vi "Brk_Pt_PRF.vi"(0 "Motion Settings In":T1={"No Motion?"=FALSE, "Motion System"=enum."NI 735x", "Motion Bd ID"=1, "Motion Profile"="SMAC1", "# Axis"=1, "Reverse Z axis?"=TRUE, "SMAC Axis"=0, "scan pair"=enum."y-(x) scan", "RT fps"=6.0, "Steps per mm"=[1000, 1000, 1000, 1000], "Motor Parameters"={"velocity ct/s"=[10000.0, 10000.0, 10000.0, 50000.0], "accel ct/s^2"=[50000.0, 50000.0, 50000.0, 200000.0]}, "One Way Scan"=FALSE, "Reverse One Way Scan"=FALSE, "Global Position (mm)"=[], "Plane"=0, "Distance between\nscan lines (um)"=0.0, "Distance between\nscan planes (um)"=0.0, "number of scan planes"=1, "Total steps in line"=0, "Xtra plane\ndistance  (um)"=100, "Xtra planes "=1, "Add Axis"=FALSE, "overshoot cts"=200, "BKPT Shift"=0, "Scan Start Time (ms)"=0, "ESP VISA"="GPIB::1::INSTR", "3rd Axis"=1, "GL Ref Out"=refnum, "Galil Address"=""} {"3rd Axis" items=["x", "y", "z", "w"]; "Xtra planes" min=1; "Xtra plane\ndistance  (um)" min=0; "Distance between\nscan planes (um)" format="%.2f"; "Distance between\nscan lines (um)" format="%.2f"; "SMAC Axis" items=["None"=0, "Axis 1"=1, "Axis 2"=2, "Axis 3"=3, "Axis 4"=4, "Axis 5"=5, "Axis 6"=6, "Axis 7"=7, "Axis 8"=8, "Vector Space 1"=17, "Vector Space 2"=18, "Vector Space 3"=19, "Vector Space 4"=20]; "Motion Bd ID" min=1 max=32 step=1}, 1 "Axis":u16(ring)=1 items=["Axis 1"=1, "Axis 2"=2, "Axis 3"=3, "Axis 4"=4, "Axis 5"=5, "Axis 6"=6, "Axis 7"=7, "Axis 8"=8], 2 "Reverse ?":bool, 11 "error in (no error)":errorcluster, 13 "Offset":i32) -> (4 "Start Position":i32, 6 "End Position":i32, 10 "Motion error":bool)   [LabVIEW 2022 SP3]
doc: "EXAMPLE: DO_WHILE Loop (Onboard Programming Template)\n\nSUMMARY:\nThis FlexMotion example demonstrates the implementation of a DO_WHILE loop data structure in an onboard program. The C equivalent of the data structure implemented here is:\n\ndo {\n// code to be repeated\nloopVar = loopVar - increment;\n} while (loopVar != 0);\n\nTHEORY OF OPERATION:\nThe flow of the DO_WHILE loop data structure goes as follows:\n(1) Program storage is begun.\n(2) The DO_WHILE loop is set up. (Loop Variable and Increment are each defined and initialized.)\n(3) A code delimiter is set using label #1.\n(4) Code to be executed each time through loop is run (in the template program, the loop variable is decremented).\n(5) The loop variable or other test condition is checked.\n(6) If the test condition is true, then we jump back to label #1. Otherwise, the condition is false so the loop terminates.\n(7) Program storage is ended.\n\nDEVELOPMENT DETAILS:\nApplication Software: LabVIEW 5.0.x\nHardware: FlexMotion controller\nDriver Software: FlexMotion Software 4.0\n\nREQUIRED HARDWARE:\n(controller only)\n\nINSTRUCTIONS:\n(0) Initialize the FlexMotion controller before running this VI. \n(1) Add the FlexMotion functions you want to execute into the block diagram where noted.\n(2) Run the VI to store the program. (The program will not be executed at this time.)\n(3) You can then run the program you have stored by calling the run_prog.flx function with the appropriate program number.\n\nADDITIONAL NOTES:\n(a) You should read the following items before writing FlexMotion onboard programs:\n(1) The Onboard Programs section of the FlexMotion Hardware User Manual (page 4-9 in the November 1998 edition).\n(2) The section about onboard variables in your FlexMotion Software Reference Manual (pages 4-11 and 4-12 in the November 1998 edition)\n(3) You will find the chapter of the FlexMotion Software Reference Manual concerning the Onboard Programming functions to be an invaluable reference resource (Chapter 12 of the November 1998 edition) along with the online help for the VI functions.\n(b) This template repeats the DO_WHILE loop as long as an expression with a variable evaluates to be true. However, you may evaluate other conditions such as move complete status instead.\n\n*NOTE: This example is not supported on the 7334 controller."
uses:
  MotionParameters.ctl
  MotionSys.ctl
  -MotionRoutines/ScanAxis.ctl
  -MotionRoutines/3rdAxis.ctl
  <vilib>/Motion/FlexMotion/FunctionsVIs/Trajectory.llb/Load Acceleration/Deceleration.flx
  <vilib>/Motion/FlexMotion/FunctionsVIs/StartStopMotion.llb/Start Motion (8 axes).flx
  <vilib>/Motion/FlexMotion/FunctionsVIs/Trajectory.llb/Wait for Move Complete (8 axes).flx
  Pulsers/PulserGlobals.vi
panel:
  out "Motion stop loop":i32
  # "Doesn't seem to work. Too much overhead to maintain PRF"
  # "1-D and 2-D B scan settings"
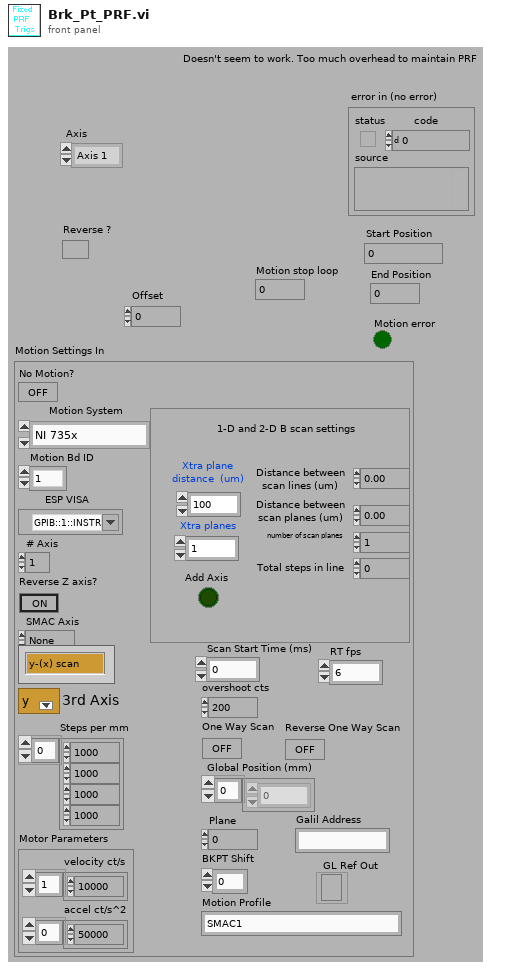
[diagram p1: front panel]
types:
  T1 = typedef "MotionParameters.ctl" = cluster{"No Motion?":bool, "Motion System":T2, "Motion Bd ID":u8, "Motion Profile":string, "# Axis":i8, "Reverse Z axis?":bool, "SMAC Axis":u16, "scan pair":T3, "RT fps":sgl, "Steps per mm":i32[], "Motor Parameters":cluster{"velocity ct/s":dbl[], "accel ct/s^2":dbl[]}, "One Way Scan":bool, "Reverse One Way Scan":bool, "Global Position (mm)":dbl[], "Plane":i32, "Distance between\nscan lines (um)":sgl, "Distance between\nscan planes (um)":sgl, "number of scan planes":i32, "Total steps in line":i32, "Xtra plane\ndistance  (um)":i32, "Xtra planes ":i32, "Add Axis":bool, "overshoot cts":i32, "BKPT Shift":i32, "Scan Start Time (ms)":u32, "ESP VISA":refnum<visa-resource-name>, "3rd Axis":T4, "GL Ref Out":refnum<k7>, "Galil Address":string}
  T2 = typedef "MotionSys.ctl" = enum16{"MM3000", "NI 735x", "Newport ESP", "No Motion Card", "Galil"}
  T3 = typedef "ScanAxis.ctl" = enum16{"y-(x) scan", "x-(y) scan", "z-(x) scan", "z-(y) scan", "y-(z) scan", "x-(z) scan", "w-(x) scan", "w-(y) scan", "w-(z) scan", "x-(w) scan", "y-(w) scan", "z-(w) scan"}
  T4 = typedef "3rdAxis.ctl" = u16
  T5 = typedef "Resource Out (Enum).flx" = u16
  T6 = typedef "Bd Id Out" = u8
  T7 = enum16{"Less Than", "Equal", "Less Than Or Equal", "Greater Than", "Not Equal", "Greater Than Or Equal", "True", "Home Found", "Index Found", "High Speed Capture", "Position Breakpoint", "Reserved", "Velocity Threshold", "Move Complete", "Profile Complete", "Blend Complete", "Motor Off", "Home Input Active", "Limit Input Active", "Software Limit Active", "Program Complete", "IO Port Match"}
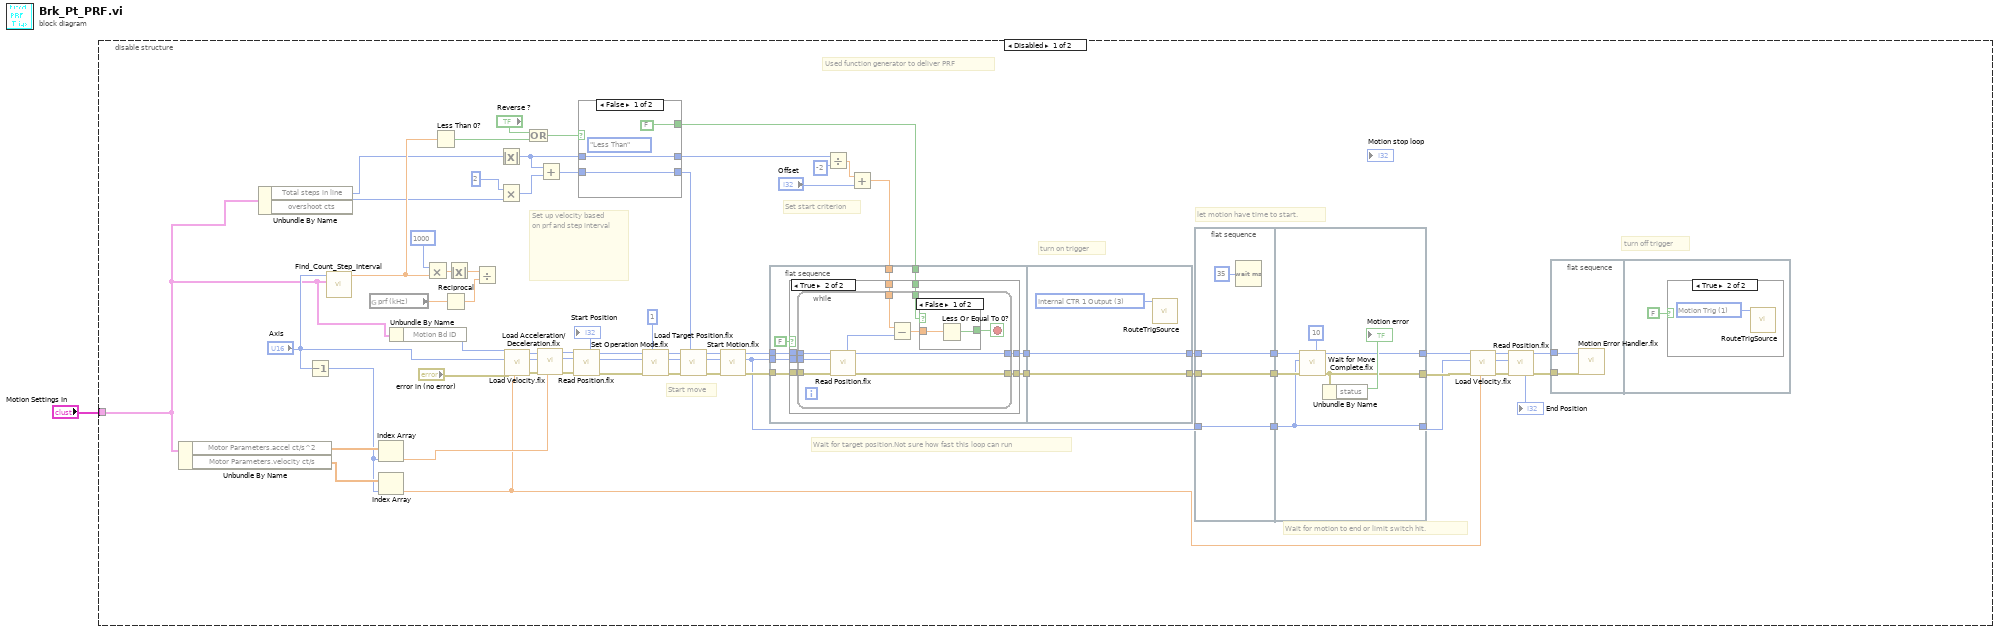
[diagram p0: block diagram]
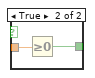
[diagram p4: hidden frame]
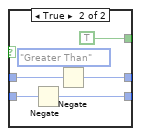
[diagram p5: hidden frame]
diagram:
  n1 = disable-structure shown="Disabled" {
    disable-tunnel: "Motion Settings In" -> [w6 _]
    frame Disabled {
      # "Wait for motion to end or limit switch hit."
      # "let motion have time to start."
      # "Used function generator to deliver PRF"
      # "turn off trigger"
      # "turn on trigger"
      # "Wait for target position.Not sure how fast this loop can run"
      # "Set start criterion"
      # "Set up velocity based on prf and step interval"
      # "Start move"
      n2 = Unbundle By Name(w6) -> ("Motor Parameters.accel ct/s^2"=w13:dbl[], "Motor Parameters.velocity ct/s"=w11:dbl[])
      n3 = Unbundle By Name(w6) -> ("Total steps in line"=w4:i32, "overshoot cts"=w7:i32)
      n4 = Decrement(x="Axis") -> (x-1=w10:u16)
      n5 = call "Find_Count_Step_Interval.vi"("Motion Settings In"=w6, "Axis"="Axis") -> ("BP Interval"=w8:dbl)  [unwired: 8 in, 1 out]
      n6 = global read "PulserGlobals.vi" "prf (kHz)"() -> (w3:dbl)
      n7 = Index Array(array=w13, index=w10) -> (element=w12:dbl)
      n8 = Index Array(array=w11, index=w10) -> (element=w2:dbl)
      n9 = Unbundle By Name(w6) -> ("Motion Bd ID"=w5:u8)
      n10 = Multiply(x=1000, y=w8) -> (x*y=w20:dbl)
      n11 = Less Than 0?(x=w8) -> (x < 0?=w57:bool)
      n12 = Reciprocal(x=w3) -> (1/x=w33:dbl)
      n13 = Absolute Value(x=w20) -> (abs(x)=w43:dbl)
      n14 = Divide(x=w43, y=w33) -> ()  [unwired: 1 out]
      n15 = Absolute Value(x=w4) -> (abs(x)=w42:i32)
      n16 = Multiply(x=2, y=w7) -> (x*y=w16:i32)
      n17 = call <vilib>:"Load Velocity.flx"("Velocity (10000)"=w2, "error in (no error)"="error in (no error)", "Axis or Vector Space"="Axis", "Board ID"=w5) -> ("error out"=w52:errorcluster, "Resource Output"=w50:T5, "Bd ID Out"=w51:T6)  [unwired: 3 out]
      n18 = Or(x="Reverse ?", y=w57) -> (x .or. y?=w55:bool)
      n19 = call "Load Acceleration/Deceleration.flx"("Acceleration (100000)"=w12, "error in (no error)"=w52, "Axis or Vector Space"=w50, "Board ID"=w51) -> ("error out"=w53:errorcluster, "Resource Output"=w49:T5, "Bd ID Out"=w54:T6)  [unwired: 1 in, 2 out]
      n20 = Add(x=w42, y=w16) -> (x+y=w48:i32)
      n21 = call <vilib>:"Read Position.flx"("error in (no error)"=w53, "Axis"=w49, "Board ID"=w54) -> ("error out"=w30:errorcluster, "Resource Output"=w28:T5, "Bd ID Out"=w29:T6, "Position"=→"Start Position":i32)  [unwired: 3 out]
      n22 = case shown="False" w55 {
        tunnel: w48 -> [w120 w125]
        tunnel: [w120 w124] -> w58
        tunnel: [w119 w122] -> w37
        tunnel: w42 -> [w119 w123]
        tunnel: [FALSE TRUE] -> w25
        frame False {
          (unwired) T7."Less Than" ("Condition Code (True)")
        }
        frame True {
          (unwired) T7."Greater Than" ("Condition Code (True)")
          n23 = Negate(x=w125) -> (-x=w124:i32)
          n24 = Negate(x=w123) -> (-x=w122:i32)
        }
      }
      n25 = call <vilib>:"Set Operation Mode.flx"("Position Mode (Absolute)"=1, "error in (no error)"=w30, "Axis or Vector Space"=w28, "Board ID"=w29) -> ("error out"=w61:errorcluster, "Resource Output"=w59:T5, "Bd ID Out"=w19:T6)  [unwired: 2 out]
      n26 = call <vilib>:"Load Target Position.flx"("Target Position (0)"=w58, "error in (no error)"=w61, "Axis"=w59, "Board ID"=w19) -> ("error out"=w62:errorcluster, "Resource Output"=w63:T5, "Bd ID Out"=w18:T6)  [unwired: 3 out]
      n27 = call-poly <vilib>:"Start Motion.flx"("error in (no error)"=w62, "Axis or Vector Space"=w63, "Board ID"=w18) -> ("error out"=w27:errorcluster, "Resource Output"=w15:T5, "Bd ID Out"=w31:T6)  [unwired: 1 in, 2 out]
      n28 = flat-sequence {
        tunnel: w31 -> [w90]
        tunnel: w27 -> [w89]
        tunnel: w26 -> [w88]
        tunnel: w25 -> [w87]
        tunnel: w15 -> [w86]
        tunnel: [w91] -> w68
        tunnel: [w85] -> w67
        tunnel: [w116] -> w24
        tunnel: [w117] -> w36
        tunnel: w68 -> [w117]
        tunnel: w67 -> [w116]
        frame #0 {
          n29 = case shown="True" FALSE {
            tunnel: [w93 w100] -> w91
            tunnel: w90 -> [w93 w99]
            tunnel: w89 -> [w92 w98]
            tunnel: w88 -> [_ w97]
            tunnel: w87 -> [_ w96]
            tunnel: w86 -> [_ w95]
            tunnel: [w92 w94] -> w85
            frame False {
            }
            frame True {
              n30 = while {
                tunnel: [w101] -> w100
                tunnel: w99 -> [w110]
                tunnel: w95 -> [w109]
                tunnel: w98 -> [w108]
                tunnel: [w107] -> w94
                tunnel: w97 -> [w105]
                tunnel: w96 -> [w102]
                stop <- w103 stop-if-true
                n31 = call <vilib>:"Read Position.flx"("error in (no error)"=w108, "Axis"=w109, "Board ID"=w110) -> ("error out"=w107:errorcluster, "Bd ID Out"=w101:T6, "Position"=w106:i32)  [unwired: 4 out]
                n32 = Subtract(x=w105, y=w106) -> (x-y=w104:dbl)
                n33 = case shown="False" w102 {
                  tunnel: w104 -> [w112 w114]
                  tunnel: [w111 w113] -> w103
                  frame False {
                    n34 = Less Or Equal To 0?(x=w112) -> (x <= 0?=w111:bool)
                  }
                  frame True {
                    n35 = Greater Or Equal To 0?(x=w114) -> (x >= 0?=w113:bool)
                  }
                }
              }
            }
          }
        }
        frame #1 {
          w115 = u16 3 items=["Function Gen Input", "Motion Trig", "Internal RT Motion Trig", "Internal CTR 1 Output"] ("Trig Source")
          n36 = call "RouteTrigSource.vi"("Trig Source"=w115) -> ()  [unwired: 10 in, 1 out]
        }
      }
      n37 = Divide(x=w37, y=-2) -> (x/y=w39:dbl)
      n38 = Add(x=w39, y="Offset") -> (x+y=w26:dbl)
      n39 = flat-sequence {
        tunnel: w36 -> [w71]
        tunnel: [w71] -> w66
        tunnel: w24 -> [w70]
        tunnel: [w70] -> w65
        tunnel: w15 -> [w69]
        tunnel: [w69] -> w64
        tunnel: w66 -> [w79]
        tunnel: w65 -> [w78]
        tunnel: [w76] -> w23
        tunnel: [w75] -> w22
        tunnel: w64 -> [w73]
        tunnel: [w73] -> w14
        frame #0 {
          n40 = Wait (ms)(milliseconds to wait=35) -> ()  [unwired: 1 out]
        }
        frame #1 {
          n41 = call-poly <vilib>:"Wait for Move Complete.flx"("Poll Interval (20 ms)"=10, "error in (no error)"=w78, "Axis or Vector Space"=w73, "Board ID"=w79) -> ("error out"=w75:errorcluster, "Bd ID Out"=w76:T6)  [unwired: 4 in, 2 out]
          n42 = Unbundle By Name(w75) -> ("status"=→"Motion error":bool)
        }
      }
      n43 = call <vilib>:"Load Velocity.flx"("Velocity (10000)"=w2, "error in (no error)"=w22, "Axis or Vector Space"=w14, "Board ID"=w23) -> ("error out"=w46:errorcluster, "Resource Output"=w45:T5, "Bd ID Out"=w47:T6)  [unwired: 3 out]
      n44 = call <vilib>:"Read Position.flx"("error in (no error)"=w46, "Axis"=w45, "Board ID"=w47) -> ("error out"=w34:errorcluster, "Bd ID Out"=w35:T6, "Position"=→"End Position":i32)  [unwired: 4 out]
      n45 = flat-sequence {
        tunnel: w35 -> [w81]
        tunnel: w34 -> [w80]
        frame #0 {
          n46 = call <vilib>:"Motion Error Handler.flx"("Board ID"=w81, "error in (no error)"=w80) -> ()  [unwired: 4 in, 10 out]
        }
        frame #1 {
          n47 = case shown="True" FALSE {
            frame False {
            }
            frame True {
              w83 = u16 1 items=["Function Gen Input", "Motion Trig", "Internal RT Motion Trig", "Internal CTR 1 Output"] ("Trig Source")
              n48 = call "RouteTrigSource.vi"("Trig Source"=w83) -> ()  [unwired: 10 in, 1 out]
            }
          }
        }
      }
    }
    frame Enabled {
    }
  }
